vi "题目5.vi"() -> ()   [LabVIEW 2017]
panel:
  in  "控制面板":T1 {"档位" scale=0.0..5.0; "油门" scale=0.0..8.0}
  out "显示面板":T2 {"油量" scale=0.0..200.0; "速度" scale=0.0..300.0; "转速" scale=0.0..8000.0}
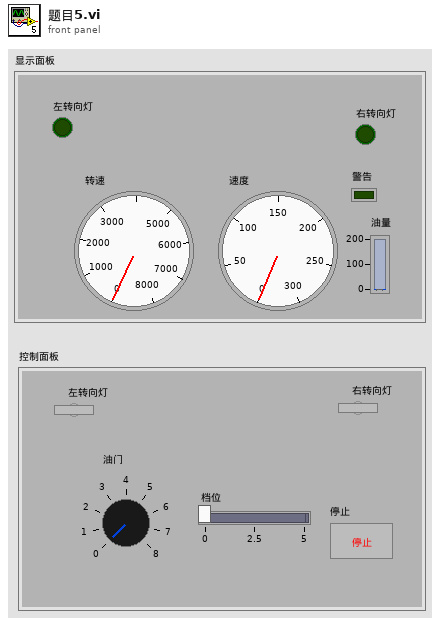
[diagram p1: front panel]
types:
  T1 = cluster{"右转向灯":bool, "油门":dbl, "档位":dbl, "停止":bool, "左转向灯":bool}
  T2 = cluster{"转速":dbl, "速度":dbl, "右转向灯":bool, "左转向灯":bool, "警告":bool, "油量":dbl}
  T3 = cluster{"zs":dbl, "v":dbl, "右转向灯":bool, "左转向灯":bool, "Blinking":bool, "y":dbl}
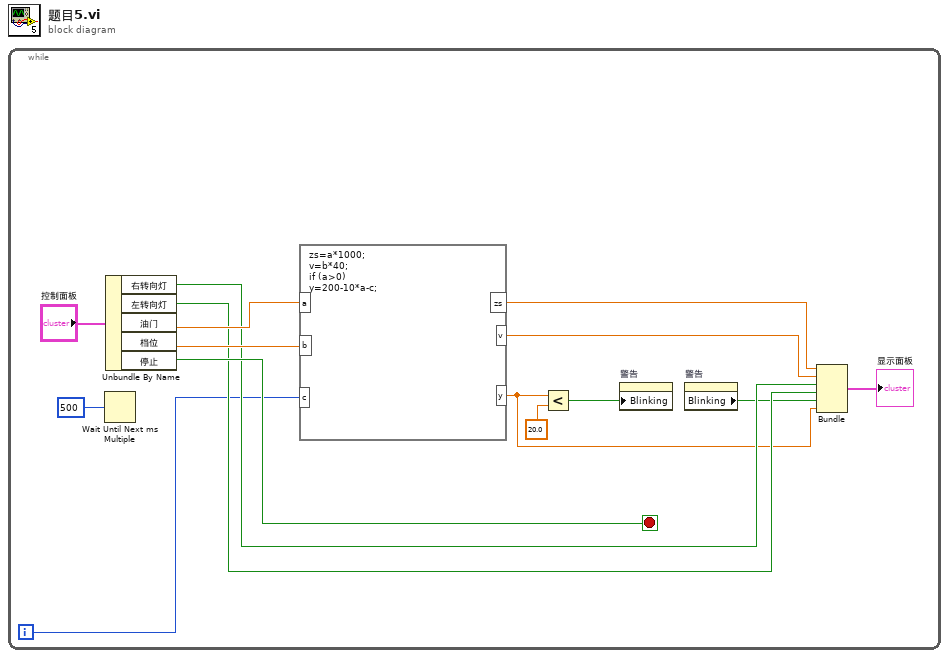
[diagram p0: block diagram]
diagram:
  n1 = while {
    i -> [w1]
    stop <- w11 stop-if-true
    n2 = Wait Until Next ms Multiple(millisecond multiple=u32 500 ("毫秒倍数")) -> ()  [unwired: 1 out]
    n3 = Unbundle By Name("控制面板") -> ("右转向灯"=w7:bool, "左转向灯"=w6:bool, "油门"=w13:dbl, "档位"=w12:dbl, "停止"=w11:bool)
    n4 = formula code="zs=a*1000;\nv=b*40;\nif (a>0)\ny=200-10*a-c;"("a"=w13, "b"=w12, "c"=w1) -> ("zs"=w9:dbl, "v"=w10:dbl, "y"=w3:dbl)
    n5 = Less?(x=w3, y=20.0) -> (x < y?=w8:bool)
    n6 = property on="警告" class="Bool (严格)"("Blinking"=w8) -> ()  [unwired: 2 in, 2 out]
    n7 = property on="警告" class="Bool (严格)"() -> ("Blinking"=w5:bool)  [unwired: 2 in, 2 out]
    n8 = Bundle("zs"=w9, "v"=w10, "右转向灯"=w7, "左转向灯"=w6, "Blinking"=w5, "y"=w3) -> (→"显示面板":T3)  [unwired: 1 in]
  }
